vi "DHE_UpdateTPNTHdr.vi"(8 "error in (no error)":errorcluster, 9 "TP value":dbl format="%.3f", 10 "TP name":string, 11 "Database RefNum in":T1) -> (0 "error out":errorcluster)   [LabVIEW 2016]
uses:
  DBSHAND/private/vis/DatabaseHand_RefNum.ctl
  DBSHAND/private/vis/DatabaseHand_Element_Set(2DArr).vi
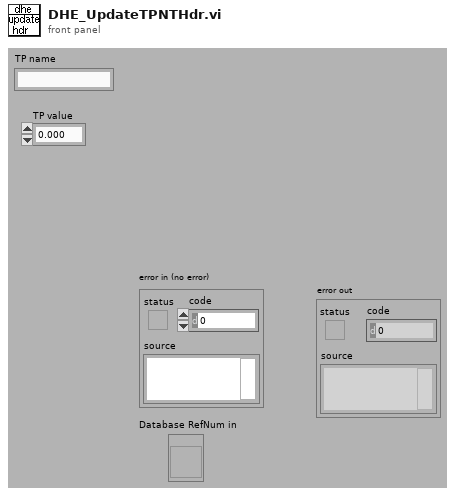
[diagram p1: front panel]
types:
  T1 = typedef "DatabaseHand_RefNum.ctl" = refnum<vi>
  T2 = enum16{"read from file", "clear", "get all", "set all"}
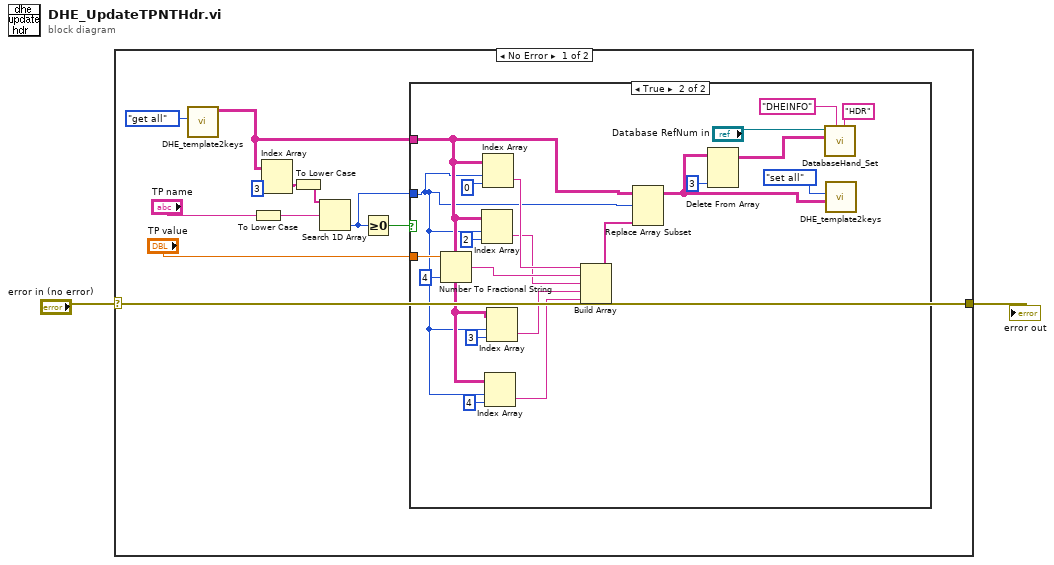
[diagram p0: block diagram]
diagram:
  n1 = case shown="No Error" "error in (no error)" {
    selector: "error in (no error)" -> [w5 w35]
    tunnel: [w5 w35] -> w1
    frame No Error {
      n2 = call "DHE_template2keys.vi"("Action"=enum16{"read from file", "clear", "get all"}."get all") -> ("HdrInfo"=w8:string[][])  [unwired: 3 in, 7 out]
      n3 = To Lower Case(string="TP name") -> (all lower case string=w3:string)
      n4 = Index Array(array=w8, index (col)=3 ("disabled index (col)")) -> (element=w10:string[])  [unwired: 1 in]
      n5 = To Lower Case(string=w10) -> (all lower case string=w4:string[])
      n6 = Search 1D Array(1D array=w4, element=w3) -> (index of element=w12:i32)  [unwired: 1 out]
      n7 = Greater Or Equal To 0?(x=w12) -> (x >= 0?=w13:bool)
      n8 = case shown="True" w13 {
        tunnel: w12 -> [_ w16]
        tunnel: "TP value" -> [_ w34]
        tunnel: w8 -> [_ w19]
        frame False {
        }
        frame True {
          n9 = Number To Fractional String(number=w34, precision (6)=i16 4) -> (F-format string=w22:string)  [unwired: 2 out]
          n10 = Index Array(array=w19, index (row)=w16, index (col)=2 ("disabled index (col)")) -> (element=w21:string)
          n11 = Index Array(array=w19, index (row)=w16, index (col)=0 ("disabled index (col)")) -> (element=w23:string)
          n12 = Index Array(array=w19, index (row)=w16, index (col)=4 ("disabled index (col)")) -> (element=w18:string)
          n13 = Index Array(array=w19, index (row)=w16, index (col)=3 ("disabled index (col)")) -> (element=w27:string)
          n14 = Build Array(w23, w22, w21, w27, w18) -> (w32:string[])
          n15 = Replace Array Subset(array=w19, new element=w32, index (row)=w16) -> (w17:string[][])  [unwired: 1 in]
          n16 = Delete From Array(array=w17, index (col)=3 ("disabled index (col)")) -> (array with subset deleted=w15:string[][])  [unwired: 2 in, 1 out]
          n17 = call-poly "DatabaseHand_Set.vi"("group"="HDR", "name"="DHEINFO", "value"=w15, "Database RefNum in"="Database RefNum in") -> ()  [unwired: 4 in, 4 out]
          n18 = call "DHE_template2keys.vi"("HdrInfo In"=w17, "Action"=T2."set all") -> ()  [unwired: 2 in, 8 out]
        }
      }
    }
    frame Error {
    }
  }
  "error out" <- w1
